vi "App From Array.vi"(1 "Projects":u16, 2 "All Projects":T1[](array[typedef])) -> (0 "App Info":T1)   [LabVIEW 2018, in "Bookmark Manager.lvlib"]
uses:
  Bookmark Manager.lvlib
  <vilib>/addons/analyzer/_analyzerctrls.llb/VIAnCtl Analysis App Info.ctl
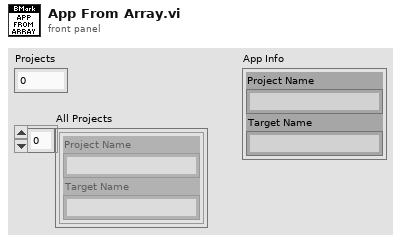
[diagram p1: front panel]
types:
  T1 = typedef "VIAnCtl Analysis App Info.ctl" = cluster{"Project Name":string, "Target Name":string}
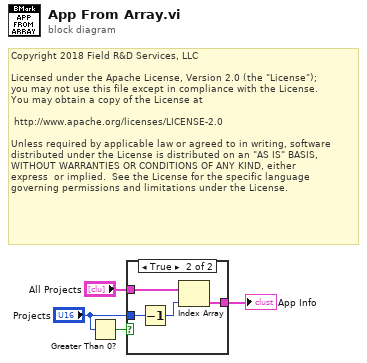
[diagram p0: block diagram]
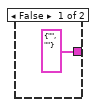
[diagram p2: hidden frame]
diagram:
  # "Copyright 2018 Field R&D Services, LLC\n\nLicensed under the Apache License, Version 2.0 (the \"License\");\nyou may not use this file except in compliance with the License.\nYou may obtain a copy of the License at\n\n\thttp://www.apache.org/licenses/LICENSE-2.0\n\nUnless required by applicable law or agreed to in writing, software\ndistributed under the License is distributed on an \"AS IS\" BASIS,\nWITHOUT WARRANTIES OR CONDITIONS OF ANY KIND, either \nexpress  or implied.  See the License for the specific language \ngoverning permissions and limitations under the License."
  n1 = Greater Than 0?(x="Projects") -> (x > 0?=w3:bool)
  n2 = case shown="True" w3 {
    tunnel: "All Projects" -> [_ w9]
    tunnel: "Projects" -> [_ w8]
    tunnel: [T1 {"Project Name"="", "Target Name"=""} ("App Info") w6] -> w4
    frame False {
    }
    frame True {
      n3 = Decrement(x=w8) -> (x-1=w7:u16)
      n4 = Index Array(array=w9, index=w7) -> (element=w6:T1)
    }
  }
  "App Info" <- w4
